vi "Connect to Keyboard.vi"() -> (4 "key info":T1(array[cluster]), 10 "device ID":refnum<k1>, 15 "error out":errorcluster)   [LabVIEW 2014]
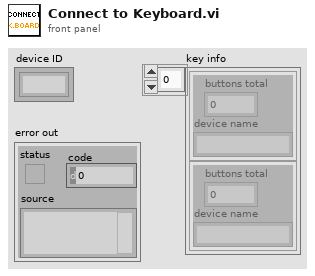
[diagram p1: front panel]
types:
  T1 = cluster{"buttons total":u32, "device name":string}[]
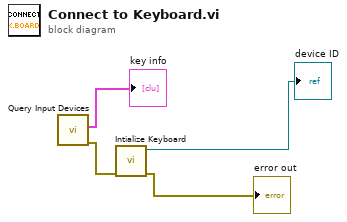
[diagram p0: block diagram]
diagram:
  n1 = call <vilib>:"Query Input Devices.vi"() -> ("error out"=w2:errorcluster, "key info"=→"key info":T1)  [unwired: 8 in, 2 out]
  n2 = call <vilib>:"Intialize Keyboard.vi"("error in (no error)"=w2) -> ("error out"=→"error out":errorcluster, "device ID"=→"device ID":refnum<k1>)  [unwired: 9 in]
